vi "Do.vi"(8 "error in (no error)":errorcluster, 10 "Actor in":refnum<class "Actor.lvclass">, 11 "Manual EMS Msg":refnum<class "Manual EMS Msg.lvclass">) -> (0 "error out":errorcluster, 2 "Actor out":refnum<class "Actor.lvclass">)   [LabVIEW 2018, in "EMS User Interface Actor.lvlib" / "Manual EMS Msg.lvclass"]
doc: "This VI delivers the message to the actor by calling the appropriate method(s) on the actor."
uses:
  Manual EMS Msg.lvclass
  <vilib>/ActorFramework/Actor/Actor.lvclass
  EMS User Interface/EMS User Interface.lvclass
  C:/Program Files (x86)/National Instruments/LabVIEW 2018/vi.lib/ActorFramework/Actor/Actor.lvclass
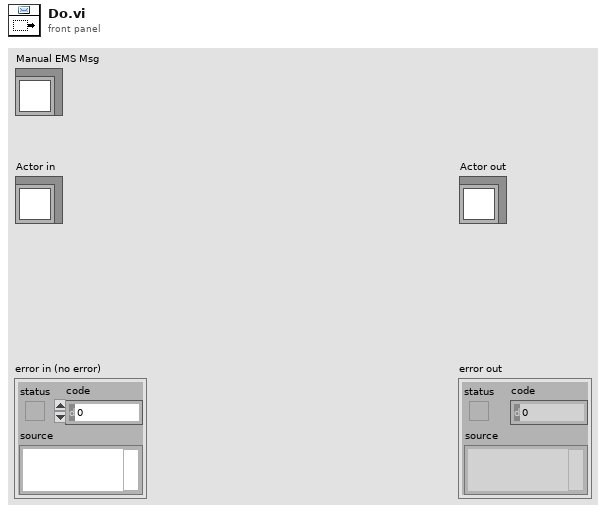
[diagram p1: front panel]
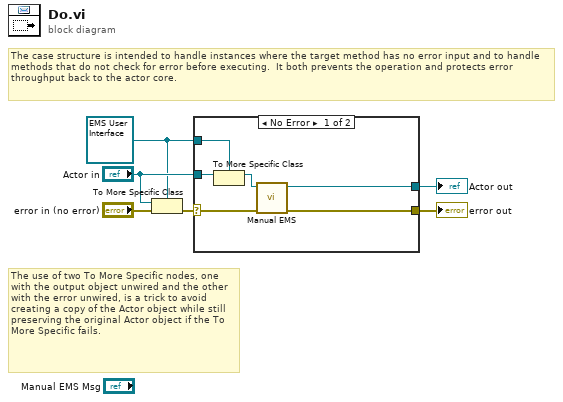
[diagram p0: block diagram]
diagram:
  w2 = refnum<class "EMS User Interface.lvclass"> refnum ("Actor in")
  # "The use of two To More Specific nodes, one with the output object unwired and the other with the error unwired, is a trick to avoid creating a copy of the Actor object while still preserving the original Actor object if the To More Specific fails."
  # "The case structure is intended to handle instances where the target method has no error input and to handle methods that do not check for error before executing.  It both prevents the operation and protects error throughput back to the actor core."
  n1 = To More Specific Class(target class=w2, reference="Actor in", error in="error in (no error)") -> (error out=w1:errorcluster)  [unwired: 1 out]
  n2 = case shown="No Error" w1 {
    selector: w1 -> [w10 w14]
    tunnel: [w12 w14] -> w6
    tunnel: [w11 w13] -> w5
    tunnel: "Actor in" -> [w9 w13]
    tunnel: w2 -> [w8 _]
    frame No Error {
      n3 = To More Specific Class(target class=w8, reference=w9) -> (specific class reference=w7:refnum<class "EMS User Interface.lvclass">)  [unwired: 1 in, 1 out]
      n4 = call "Manual EMS.vi"("error in"=w10, "Master Controller in"=w7) -> ("error out"=w12:errorcluster, "dup Master Controller out"=w11:refnum<class "EMS User Interface.lvclass">)  [unwired: 8 in]
    }
    frame Error {
      # "If type check fails, pass the original object out again."
    }
  }
  "error out" <- w6
  "Actor out" <- w5
